vi "Application By Target.vi"(8 "Error In":errorcluster, 10 "Target Name":string, 11 "Project In":refnum<vi>) -> (0 "Error Out":errorcluster, 2 "App":refnum<vi>, 3 "Project Out":refnum<vi>)   [LabVIEW 2018, in "Bookmark Manager.lvlib"]
uses:
  Bookmark Manager.lvlib
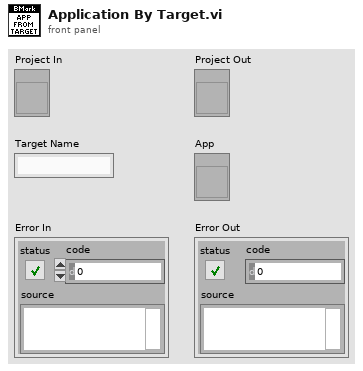
[diagram p1: front panel]
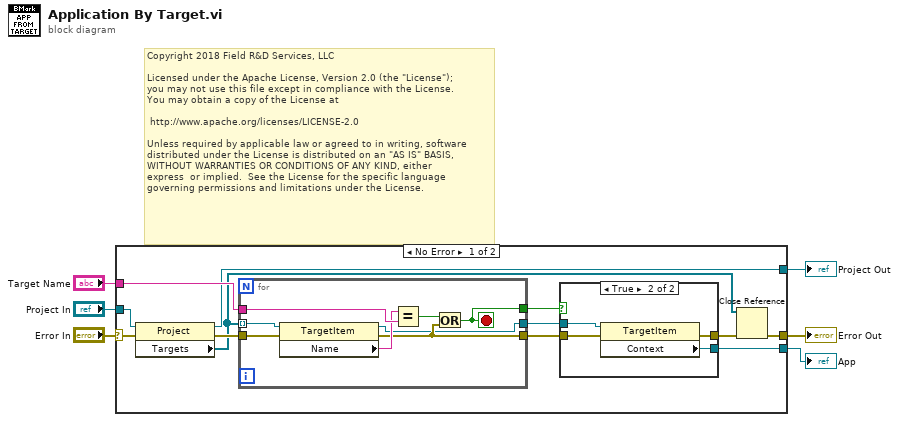
[diagram p0: block diagram]
diagram:
  # "Copyright 2018 Field R&D Services, LLC\n\nLicensed under the Apache License, Version 2.0 (the \"License\");\nyou may not use this file except in compliance with the License.\nYou may obtain a copy of the License at\n\n\thttp://www.apache.org/licenses/LICENSE-2.0\n\nUnless required by applicable law or agreed to in writing, software\ndistributed under the License is distributed on an \"AS IS\" BASIS,\nWITHOUT WARRANTIES OR CONDITIONS OF ANY KIND, either \nexpress  or implied.  See the License for the specific language \ngoverning permissions and limitations under the License."
  n1 = case shown="No Error" "Error In" {
    selector: "Error In" -> [w16 w33]
    tunnel: "Target Name" -> [w17 _]
    tunnel: [w9 w33] -> w5
    tunnel: "Project In" -> [w15 w32]
    tunnel: [w12 _] -> w2
    tunnel: [w7 w32] -> w1
    frame No Error {
      n2 = property class="Project"(reference=w15, error in=w16) -> (reference out=w7:refnum<vi>, error out=w18:errorcluster, "Targets"=w8:refnum<vi>[])
      n3 = for {
        tunnel: w18 -> [w31]
        tunnel: w8 -> [w29] mode=indexing
        tunnel: w17 -> [w30]
        tunnel: [w27] -> w11
        tunnel: [w26] -> w14
        tunnel: [w24] -> w13
        stop <- w26 stop-if-true
        n4 = property class="TargetItem"(reference=w29, error in=w31) -> (reference out=w24:refnum<vi>, error out=w27:errorcluster, "Name"=w28:string)
        n5 = Equal?(x=w28, y=w30) -> (x = y?=w25:bool)
        n6 = Or(x=w25, y=w27) -> (x .or. y?=w26:bool)
      }
      n7 = case shown="True" w14 {
        tunnel: w13 -> [_ w23]
        tunnel: [_ w22] -> w12
        tunnel: w11 -> [w19 w21]
        tunnel: [w19 w20] -> w10
        frame False {
        }
        frame True {
          n8 = property class="TargetItem"(reference=w23, error in=w21) -> (error out=w20:errorcluster, "Context"=w22:refnum<vi>)  [unwired: 1 out]
        }
      }
      n9 = Close Reference(reference=w8, error in (no error)=w10) -> (error out=w9:errorcluster)
    }
    frame Error {
    }
  }
  "Error Out" <- w5
  "App" <- w2
  "Project Out" <- w1
